vi "Read Formated Parameters.vi"(8 "error in (no error)":errorcluster, 11 "Mag Lab Parameters in":refnum<class "Mag Lab Parameters.lvclass">) -> (0 "error out":errorcluster, 2 "Formated parameters":string, 3 "Mag Lab Parameters out":refnum<class "Mag Lab Parameters.lvclass">)   [LabVIEW 2015, in "Mag Lab Parameters.lvclass"]
uses:
  Mag Lab Parameters.lvclass
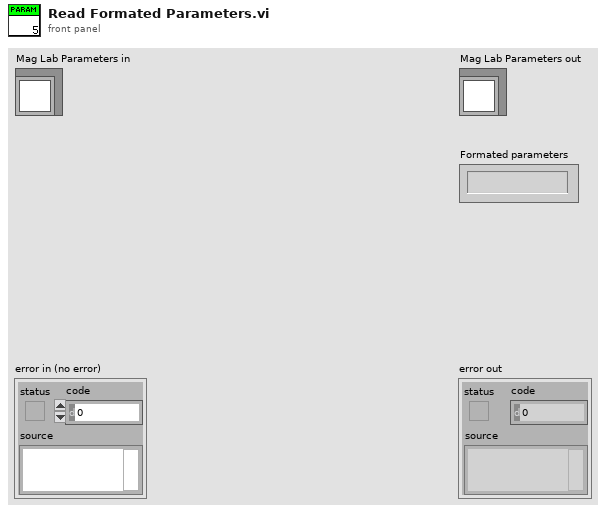
[diagram p1: front panel]
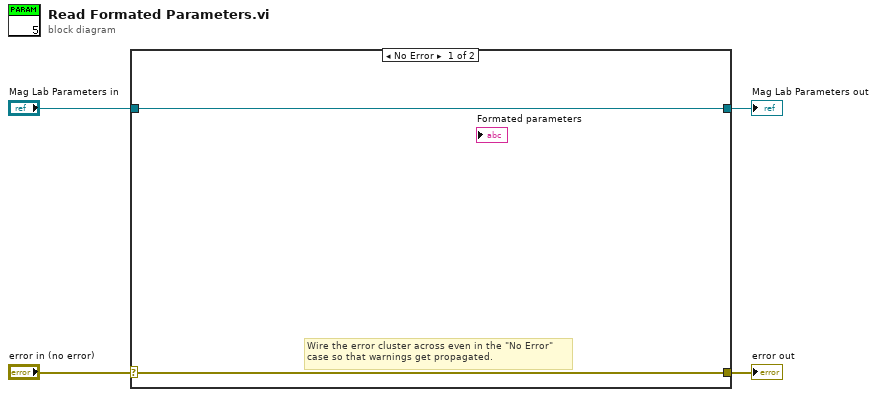
[diagram p0: block diagram]
diagram:
  n1 = case shown="No Error" "error in (no error)" {
    selector: "error in (no error)" -> [w5 w8]
    tunnel: [w5 w8] -> w3
    tunnel: [w6 w7] -> w1
    tunnel: "Mag Lab Parameters in" -> [w6 w7]
    frame No Error {
      # "Wire the error cluster across even in the \"No Error\"\ncase so that warnings get propagated."
    }
    frame Error {
    }
  }
  "error out" <- w3
  "Mag Lab Parameters out" <- w1
